vi "Stop RFSG.vi"(8 "error in (no error)":errorcluster, 11 "RFSG Reference In":refnum<k15>) -> (0 "error out":errorcluster)   [LabVIEW 2021]
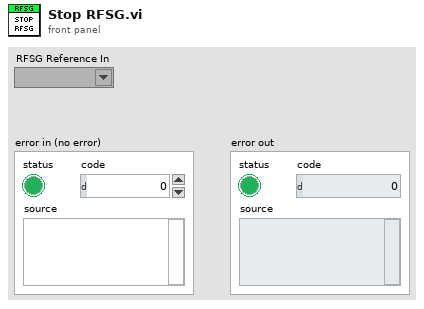
[diagram p1: front panel]
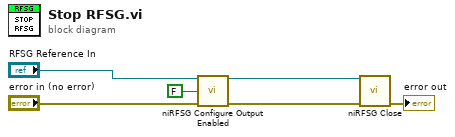
[diagram p0: block diagram]
diagram:
  n1 = call <instrlib>:"niRFSG Configure Output Enabled.vi"("instrument handle"="RFSG Reference In", "output enabled"=FALSE ("output enable"), "error in"="error in (no error)") -> ("instrument handle out"=w1:refnum<k15>, "error out"=w3:errorcluster)  [unwired: 11 in]
  n2 = call <instrlib>:"niRFSG Close.vi"("instrument handle"=w1, "error in"=w3) -> ("error out"=→"error out":errorcluster)  [unwired: 13 in]
